vi "main.vi"() -> ()   [LabVIEW 2024]
uses:
  kontrakt.ctl
  <vilib>/addons/_JKI.lib/REST Client/classes/REST Client/REST Client.lvclass
  measure_data.ctl
panel:
  in  "auto read":bool
  out "Waveform Graph 2":dbl[](graph)
  in  "Base URL":string
  in  "connect":bool
  in  "measure":bool
  in  "exit":bool
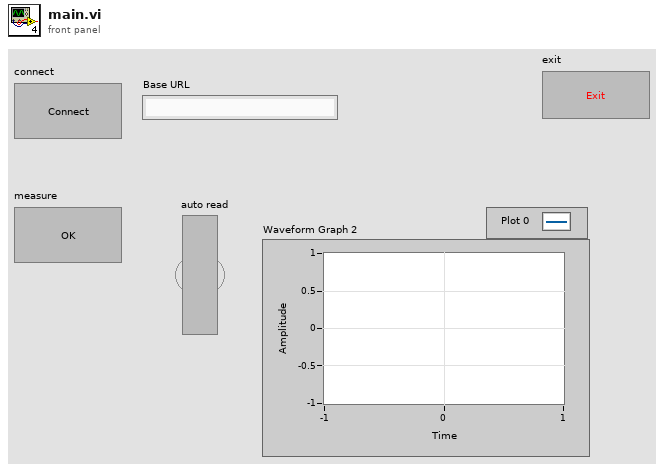
[diagram p1: front panel]
types:
  T1 = cluster{"polaczenie":refnum<class "REST Client.lvclass">, "dane":dbl[], "flag":bool, "text":string}
  T2 = typedef "kontrakt.ctl" = cluster{"akcja":enum16{"get_measure", "exit_program", "init_session", "close_session", "set_flag"}, "parametry":variant}
  T3 = enum16{"get_measure", "exit_program", "init_session", "close_session", "set_flag"}
  T4 = typedef "measure_data.ctl" = cluster{"name":string, "value":dbl, "device_id":string}
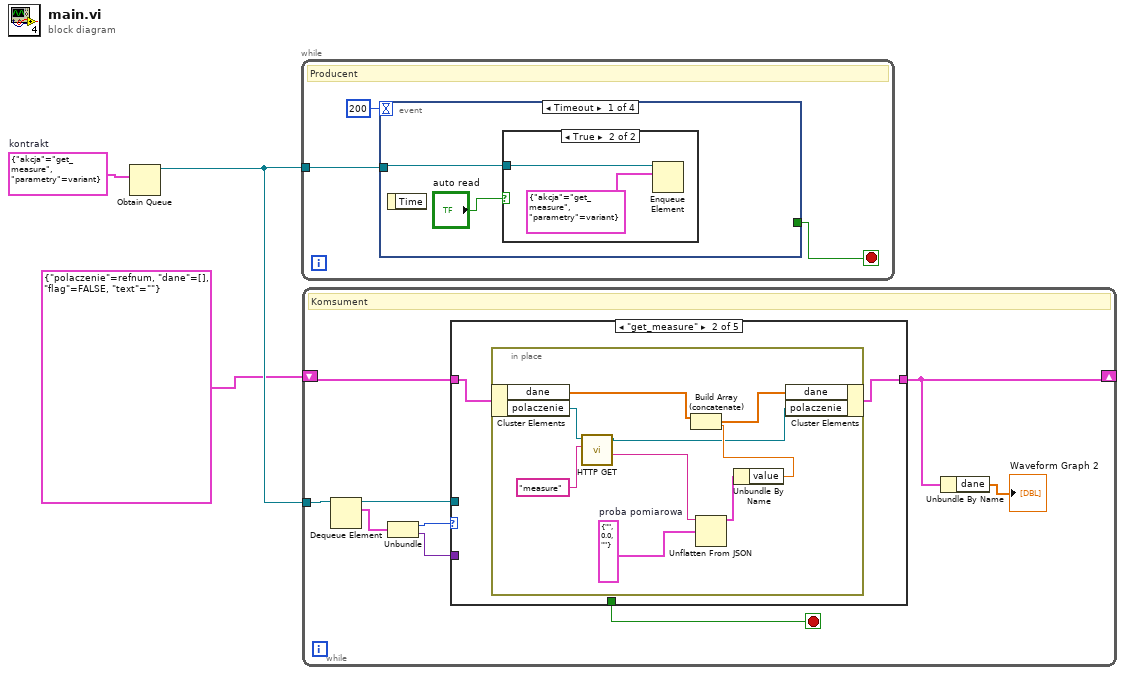
[diagram p0: block diagram]
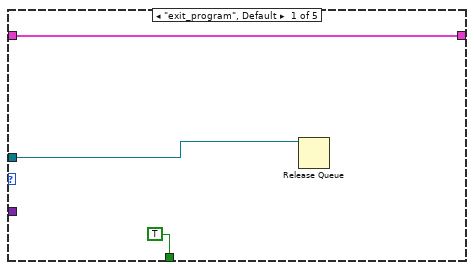
[diagram p2: hidden frame]
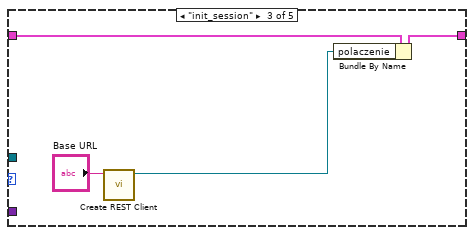
[diagram p3: hidden frame]
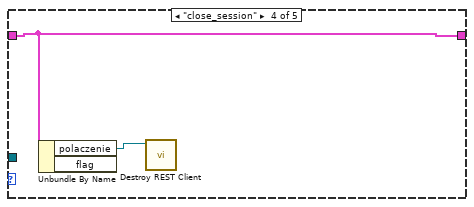
[diagram p4: hidden frame]
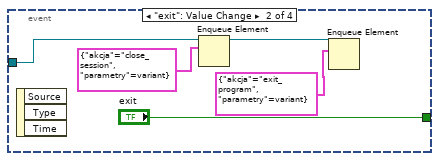
[diagram p7: hidden frame]
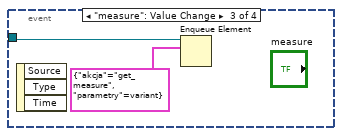
[diagram p8: hidden frame]
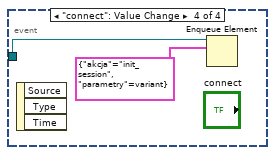
[diagram p9: hidden frame]
diagram:
  w2 = T2 {"akcja"=enum."get_measure", "parametry"=variant}  # kontrakt
  n1 = Obtain Queue(element data type=w2) -> (queue out=w3:refnum<queue>)  [unwired: 4 in, 2 out]
  n2 = while {
    tunnel: w3 -> [w6]
    stop <- w5 stop-if-true
    # "Producent"
    n3 = event shown="[0] Timeout" {
      selector: _ -> [_ _ _ _]
      dyn-events: _ -> [_ _ _ _]
      timeout: 200 -> [_ _ _ _]
      tunnel: w6 -> [w8 w14 w17 w19]
      tunnel: [_ "exit" _ _] -> w5
      event Timeout {
        n4 = event-data() -> ()  [unwired: 1 in, 1 out]
        n5 = case shown="True" "auto read" {
          tunnel: w8 -> [_ w10]
          frame False {
          }
          frame True {
            n6 = Enqueue Element(queue=w10, element=T2 {"akcja"=enum."get_measure", "parametry"=variant}) -> ()  [unwired: 2 in, 3 out]
          }
        }
      }
      event "exit": Value Change {
        n7 = event-data() -> ()  [unwired: 1 in, 3 out]
        n8 = Enqueue Element(queue=w14, element=T2 {"akcja"=enum."close_session", "parametry"=variant}) -> (queue out=w12:refnum<queue>)  [unwired: 2 in, 2 out]
        n9 = Enqueue Element(queue=w12, element=T2 {"akcja"=enum."exit_program", "parametry"=variant}) -> ()  [unwired: 2 in, 3 out]
      }
      event "measure": Value Change {
        n10 = event-data() -> ()  [unwired: 1 in, 3 out]
        n11 = Enqueue Element(queue=w17, element=T2 {"akcja"=enum."get_measure", "parametry"=variant}) -> ()  [unwired: 2 in, 3 out]
      }
      event "connect": Value Change {
        n12 = event-data() -> ()  [unwired: 1 in, 3 out]
        n13 = Enqueue Element(queue=w19, element=T2 {"akcja"=enum."init_session", "parametry"=variant}) -> ()  [unwired: 2 in, 3 out]
      }
    }
  }
  n14 = while {
    tunnel: w3 -> [w28]
    shift-right: [w21] -> _
    shift-left: T1 {"polaczenie"=refnum, "dane"=[], "flag"=FALSE, "text"=""} -> [w22]
    stop <- w23 stop-if-true
    # "Komsument"
    n15 = Dequeue Element(queue=w28) -> (queue out=w24:refnum<queue>, element=w27:T2)  [unwired: 2 in, 2 out]
    n16 = Unbundle(w27) -> ("akcja"=w26:T3, "parametry"=w25:variant)
    n17 = case shown="\"get_measure\"" w26 {
      tunnel: w25 -> [_ _ _ _ _]
      tunnel: w24 -> [w31 _ _ _ _]
      tunnel: [TRUE _ _ _ _] -> w23
      tunnel: w22 -> [w29 w33 w45 w48 w49]
      tunnel: [w29 w32 w44 w48 w49] -> w21
      frame "exit_program", Default {
        n18 = Release Queue(queue=w31) -> ()  [unwired: 2 in, 3 out]
      }
      frame "get_measure" {
        n19 = in-place "In Place Element Structure" {
          w39 = T4 {"name"="", "value"=0.0, "device_id"=""}  # proba pomiarowa
          n20 = in-place-cluster #1(w33) -> ("dane"=w37:dbl[], "polaczenie"=w35:refnum<class "REST Client.lvclass">)
          n21 = call-dynamic "HTTP GET.vi"("Path"="measure", "REST Client in"=w35) -> ("Response body"=w42:string, "REST Client out"=w34:refnum<class "REST Client.lvclass">)  [unwired: 4 in, 4 out]
          n22 = Unflatten From JSON(JSON string=w42, type and defaults=w39) -> (value=w41:T4)  [unwired: 5 in, 1 out]
          n23 = Unbundle By Name(w41) -> ("value"=w40:dbl)
          n24 = Build Array (concatenate)(w37, w40) -> (w36:dbl[])
          n25 = in-place-cluster #1("dane"=w36, "polaczenie"=w34) -> (w32:T1)
        }
      }
      frame "init_session" {
        n26 = call <vilib>:"Create REST Client.vi"("Base URL"="Base URL") -> ("REST Client out"=w43:refnum<class "REST Client.lvclass">)  [unwired: 9 in, 1 out]
        n27 = Bundle By Name(cluster=w45, "polaczenie"=w43) -> (w44:T1)
      }
      frame "close_session" {
        n28 = Unbundle By Name(w48) -> ("polaczenie"=w47:refnum<class "REST Client.lvclass">)  [unwired: 1 out]
        n29 = call-dynamic "Destroy REST Client.vi"("REST Client in"=w47) -> ()  [unwired: 10 in, 1 out]
      }
      frame "set_flag" {
      }
    }
    n30 = Unbundle By Name(w21) -> ("dane"=→"Waveform Graph 2":dbl[])
  }
